vi "Validate_Create & Compile Functions.vi"(0 "scripts manager in":refnum<class "scripts manager.lvclass">, 5 "Functions in":T1[](array[typedef]), 11 "error in (no error)":errorcluster) -> (4 "scripts manager":refnum<class "scripts manager.lvclass">, 6 "Comiplation message":T2[](array[typedef]), 15 "error out":errorcluster)   [LabVIEW 2016, in "scripts manager.lvclass"]
uses:
  scripts manager.lvclass
  common/function utils/Validate_message.ctl
  common/function utils/Validate_MessageStatus.ctl
  common/line and indent/Line Details.ctl
  scripts manager.lvclass/scripts manager.ctl
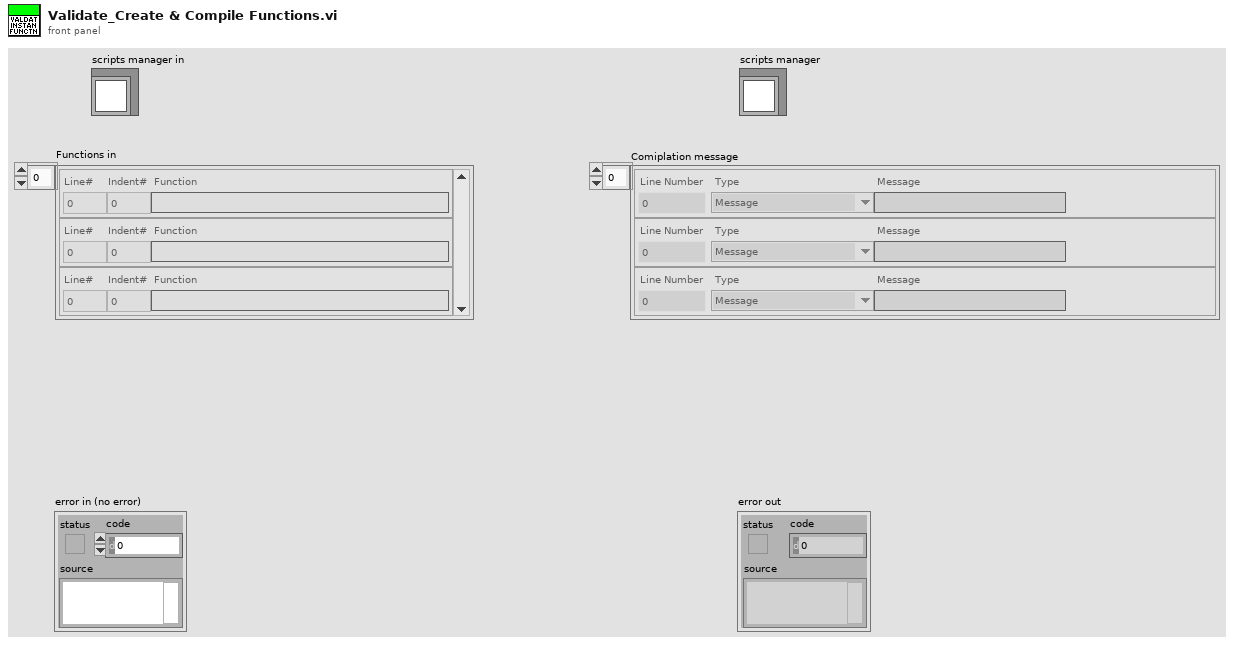
[diagram p1: front panel]
types:
  T1 = typedef "Line Details.ctl" = cluster{"Line#":i64, "Indent#":i64, "Function":string}
  T2 = typedef "Validate_message.ctl" = cluster{"Line Number":i64, "Type":T3, "Message":string}
  T3 = typedef "Validate_MessageStatus.ctl" = enum16{"Message", "Warning", "Error"}
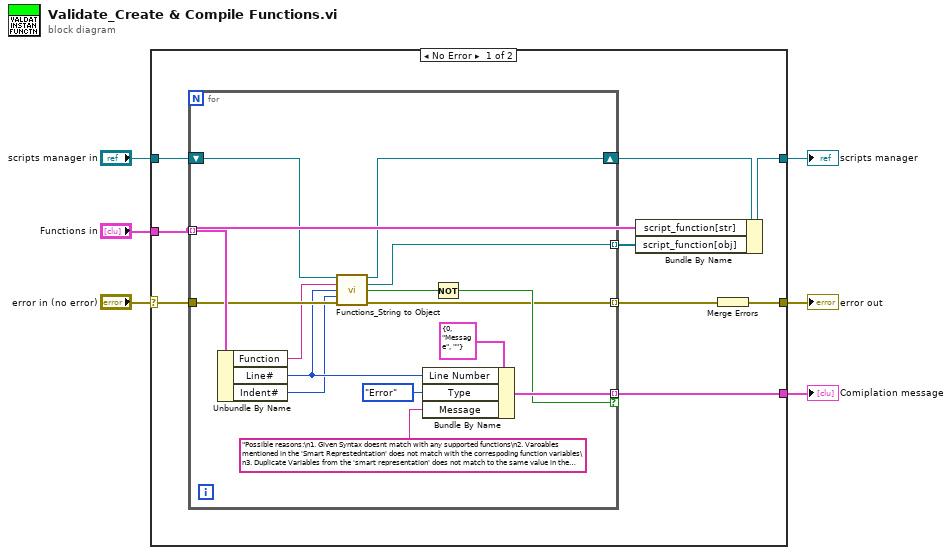
[diagram p0: block diagram]
diagram:
  n1 = case shown="No Error" "error in (no error)" {
    selector: "error in (no error)" -> [w15 w32]
    tunnel: [w13 w32] -> w5
    tunnel: [w12 _] -> w4
    tunnel: [w11 w31] -> w3
    tunnel: "scripts manager in" -> [w8 w31]
    tunnel: "Functions in" -> [w9 _]
    frame No Error {
      n2 = for {
        tunnel: w9 -> [w30] mode=indexing
        tunnel: w15 -> [w25]
        tunnel: [w21] -> w14 mode=indexing
        tunnel: [w20] -> w10 mode=indexing
        tunnel: [w28] -> w12 mode=indexing if=w27
        shift-right: [w23] -> w7
        shift-left: w8 -> [w26]
        n3 = Unbundle By Name(w30) -> ("Function"=w24:string, "Line#"=w18:i64, "Indent#"=w17:i64)
        n4 = call-dynamic "Functions_String to Object.vi"("scripts manager in"=w26, "Functions"=w24, "Line#"=w18, "Indent#"=w17, "error in (no error)"=w25) -> ("scripts manager out"=w23:refnum<class "scripts manager.lvclass">, "function obj"=w20:refnum<class "functionbase.lvclass">, "function created"=w22:bool, "error out"=w21:errorcluster)  [unwired: 7 in]
        n5 = Bundle By Name(cluster=T2 {"Line Number"=0, "Type"=enum."Message", "Message"=""} ("Message"), "Line Number"=w18, "Type"=Validate_MessageStatus."Error", "Message"="Possible reasons:\n1. Given Syntax doesnt match with any supported functions\n2. Varoables mentioned in the 'Smart Represtedntation' does not match with the correspoding function variables\n3. Duplicate Variables from the 'smart representation' does not match to the same value in the script\n4. Smart Variables does not match the Function variable data type\n5. Invalid function is represented in the script in place of a variable") -> (w28:T2)
        n6 = Not(x=w22) -> (.not. x?=w27:bool)
      }
      n7 = Bundle By Name(cluster=w7, "script_function[str]"=w9, "script_function[obj]"=w10) -> (w11:refnum<class "scripts manager.lvclass">)
      n8 = Merge Errors(w14) -> (w13:errorcluster)
    }
    frame Error {
    }
  }
  "error out" <- w5
  "Comiplation message" <- w4
  "scripts manager" <- w3
